vi "Process_15_Windows.vi"(8 "Training Completed":bool, 10 "RT FIFO not empty":bool, 11 "Non-Partitioned Data":sgl[][](array[numeric])) -> (2 "Send to NN":bool, 3 "Nr of Rows":i32)   [LabVIEW 2020]
uses:
  Pre-Processing/Number_of_Windows.vi
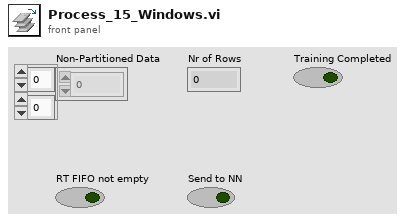
[diagram p1: front panel]
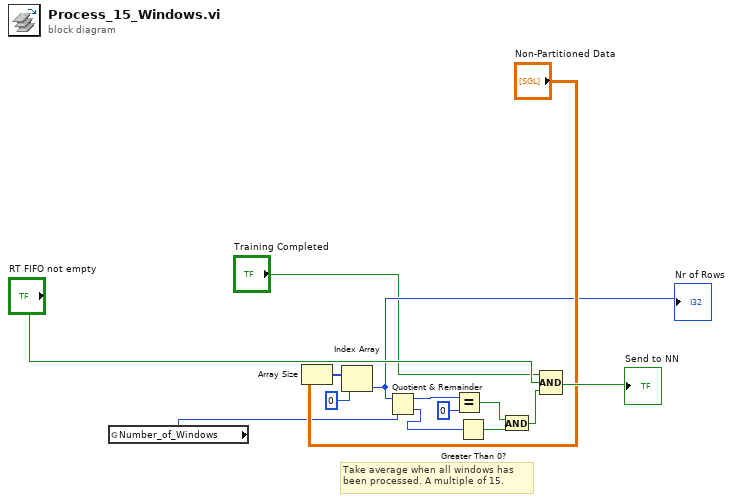
[diagram p0: block diagram]
diagram:
  # "Take average when all windows has \nbeen processed. A multiple of 15."
  n1 = global read "Number_of_Windows.vi" "Number_of_Windows"() -> (w4:i64)
  n2 = Array Size(array="Non-Partitioned Data") -> (size(s)=w2:i32[])
  n3 = Index Array(array=w2, index=0) -> (element=w6:i32)
  "Nr of Rows" <- w6
  n4 = Quotient & Remainder(x=w6, y=w4) -> (x-y*floor(x/y)=w5:i64, floor(x/y)=w10:i64)
  n5 = Equal?(x=w5, y=0) -> (x = y?=w8:bool)
  n6 = Greater Than 0?(x=w10) -> (x > 0?=w11:bool)
  n7 = And(x=w8, y=w11) -> (x .and. y?=w12:bool)
  n8 = Compound Arithmetic op=AND("Training Completed", "RT FIFO not empty", w12) -> (→"Send to NN":bool)
